vi "main_ctrl.vi"(8 "error in":errorcluster) -> (0 "error out":errorcluster caption="Error")   [LabVIEW 2013]
uses:
  <vilib>/Rock Robotics/WPI/DriverStation/WPI_DriverStationRobotMode2.ctl
  typedefs/fg_typedef.ctl
  typedefs/vision enable.ctl
  typedefs/vision data.ctl
  typedefs/subStates.ctl
  typedefs/singleUseSubstate.ctl
  <vilib>/Rock Robotics/WPI/Solenoid/WPI_SolenoidValue.ctl
  <vilib>/Rock Robotics/WPI/Compressor/WPI_CompressorGetSetRefNum.vi
  <vilib>/Rock Robotics/WPI/RobotDrive/WPI_RobotDriveGetSetRefNum.vi
  <vilib>/Rock Robotics/WPI/Solenoid/WPI_SolenoidSetEnum.vi
  <vilib>/Rock Robotics/WPI/RobotDrive/WPI_RobotDriveArcadeDrive_Standard(NoSaturation).vi
panel:
  out "Robot Mode":T1
  out "Vision SPI":u32
  out "Vision IPS":dbl
  out "Main IPS":dbl
  out "Main SPI":u32
  # "MAIN CONTROL"
  # "holds robot control code - dual parallel state machine"
  # "SPI: milliseconds per iteration\nIPS: iterations per second"
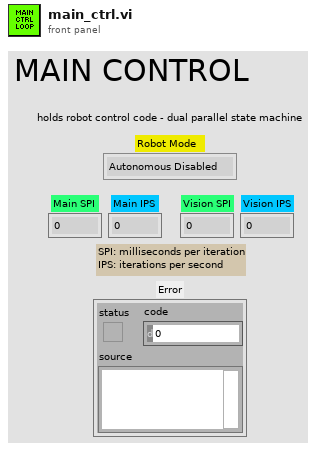
[diagram p1: front panel]
types:
  T1 = typedef "WPI_DriverStationRobotMode2.ctl" = enum16{"Autonomous Disabled", "Autonomous Enabled", "Teleop Disabled", "Teleop Enabled", "Timeout", "Finish", "Test Disabled", "Test Enabled"}
  T2 = typedef "vision data.ctl" = cluster{"x":dbl, "y":dbl, "area":dbl, "width":dbl, "height":dbl, "Hot Goal Present?":bool, "distance":dbl}
  T3 = typedef "vision enable.ctl" = enum16{"Enable", "Disable", "Stop"}
  T4 = typedef "fg_typedef.ctl" = enum16{"Get", "Set"}
  T5 = typedef "WPI_RobotDriveDevRef.ctl" = cluster{"DevStatus":errorcluster, "Motors[]":T6[], "Square Inputs":bool, "Max Output":dbl, "Isochronous":bool}
  T6 = typedef "WPI_MotorControlDeviceRef.ctl" = cluster{"DeviceStatus":errorcluster, "Type":enum16{"PWM", "CAN"}, "PWM":cluster{"Digital Module":T7, "PWM Channel":T8, "DeadBand":T9}, "CAN":cluster{"Device Number":u8, "Control Mode":T10, "Semaphore":T11, "Max Vout":dbl}, "Invert":bool, "TransformRef":T12, "InvTransformRef":T12}
  T7 = typedef "FPGA_TypedefDigitalModule.ctl" = enum16{"Digital Module 1", "Digital Module 2"}
  T8 = typedef "FPGA_DIOPWMChannel.ctl" = enum8{"PWM 1", "PWM 2", "PWM 3", "PWM 4", "PWM 5", "PWM 6", "PWM 7", "PWM 8", "PWM 9", "PWM 10", "Invalid"}
  T9 = typedef "WPI_PWMDeadband.ctl" = cluster{"Name":string, "maxPositivePwm":i32, "minPositivePwm":i32, "centerPwm":i32, "maxNegativePwm":i32, "minNegativePwm":i32, "angularRange":u16}
  T10 = typedef "WPI_CANJaguar_ControlMode.ctl" = enum8{"Percent VBus", "Current", "Speed", "Position", "Voltage"}
  T11 = typedef "Semaphore RefNum" = refnum<k1>
  T12 = typedef "WPI_PWMTransform_ConPane.ctl" = refnum<vi>
  T13 = typedef "WPI_SolenoidDevRef.ctl" = cluster{"DevStatus":errorcluster, "Solenoid Module":T14, "Forward Solenoid Channel":T15, "Reverse Solenoid Channel":T15}
  T14 = typedef "FPGA_TypedefSolenoidModule.ctl" = enum16{"Solenoid Module 1", "Solenoid Module 2"}
  T15 = typedef "WPI_SolenoidChannel.ctl" = enum8{"Solenoid 1", "Solenoid 2", "Solenoid 3", "Solenoid 4", "Solenoid 5", "Solenoid 6", "Solenoid 7", "Solenoid 8", "Invalid"}
  T16 = typedef "WPI_CompressorDevRef.ctl" = cluster{"DevStatus":errorcluster, "DigitalInputDevRef":T17, "RelayDevRef":T19}
  T17 = typedef "WPI_DigitalInputDevRef.ctl" = cluster{"DevStatus":errorcluster, "DIO Channel":T18, "Digital Module":T7}
  T18 = typedef "FPGA_DIOChannel.ctl" = enum8{"DIO 1", "DIO 2", "DIO 3", "DIO 4", "DIO 5", "DIO 6", "DIO 7", "DIO 8", "DIO 9", "DIO 10", "DIO 11", "DIO 12", "DIO 13", "DIO 14", "Invalid"}
  T19 = typedef "WPI_RelayDevRef.ctl" = cluster{"DevStatus":errorcluster, "Relay Channel":T20, "Digital Module":T7, "Relay Direction":T21}
  T20 = typedef "FPGA_DIORelayChannel.ctl" = enum8{"Relay 1", "Relay 2", "Relay 3", "Relay 4", "Relay 5", "Relay 6", "Relay 7", "Relay 8", "Invalid"}
  T21 = typedef "WPI_RelayDirection.ctl" = enum16{"Both directions", "Forward only", "Reverse only"}
  T22 = typedef "WPI_CameraDevRef.ctl" = cluster{"Camera Address":string, "CameraStatus":errorcluster, "Acquire Image Notifier":refnum<notifier>}
  T23 = typedef "IMAQ Image.ctl" = refnum<image>
  T24 = typedef "WPI_SolenoidValue.ctl" = enum16{"Off", "On", "Forward", "Reverse"}
  T25 = typedef "singleUseSubstate.ctl" = enum16{"null", "wait", "shift high", "shift low"}
  T26 = typedef "WPI_DriverStationDerivedRobotMode.ctl" = enum16{"Init", "Execute", "Stop"}
  T27 = typedef "subStates.ctl" = enum16{"null", "wait", "driver control", "auto", "manual override", "hold position", "rotate", "pickup", "pass", "load", "goto shoot", "shoot", "end"}
  T28 = typedef "Loop 2 Datatype.ctl" = cluster{"State":T27, "Waiting Loop":i32, "State to Wait For":i32, "Loop ID":i32, "Exit Value":i32, "Joystick Y":dbl, "Tune Speed":dbl}
  T29 = typedef "Loop 1 Datatype.ctl" = cluster{"State":T27, "Waiting Loop":i32, "State to Wait For":i32, "Loop ID":i32, "Exit Value":i32}
  T30 = typedef "Loop 3 Datatype.ctl" = cluster{"State":T27, "Waiting Loop":i32, "State to Wait For":i32, "Loop ID":i32, "Exit Value":i32, "Joystick Y":dbl, "Joystick Z":dbl}
  T31 = typedef "Loop 0 Datatype.ctl" = cluster{"State":T27, "Waiting Loop":i32, "State to Wait For":i32, "Loop ID":i32, "Exit Value":i32, "X Axis":dbl, "Y Axis":dbl, "Z Axis":dbl}
  T32 = typedef "Loop 4 Datatype.ctl" = cluster{"State":T27, "Waiting Loop":i32, "State to Wait For":i32, "Loop ID":i32, "Exit Value":i32}
  T33 = cluster{"Vision mSPI":u32, "Main mSPI":u32, "Dash mSPI":u32}
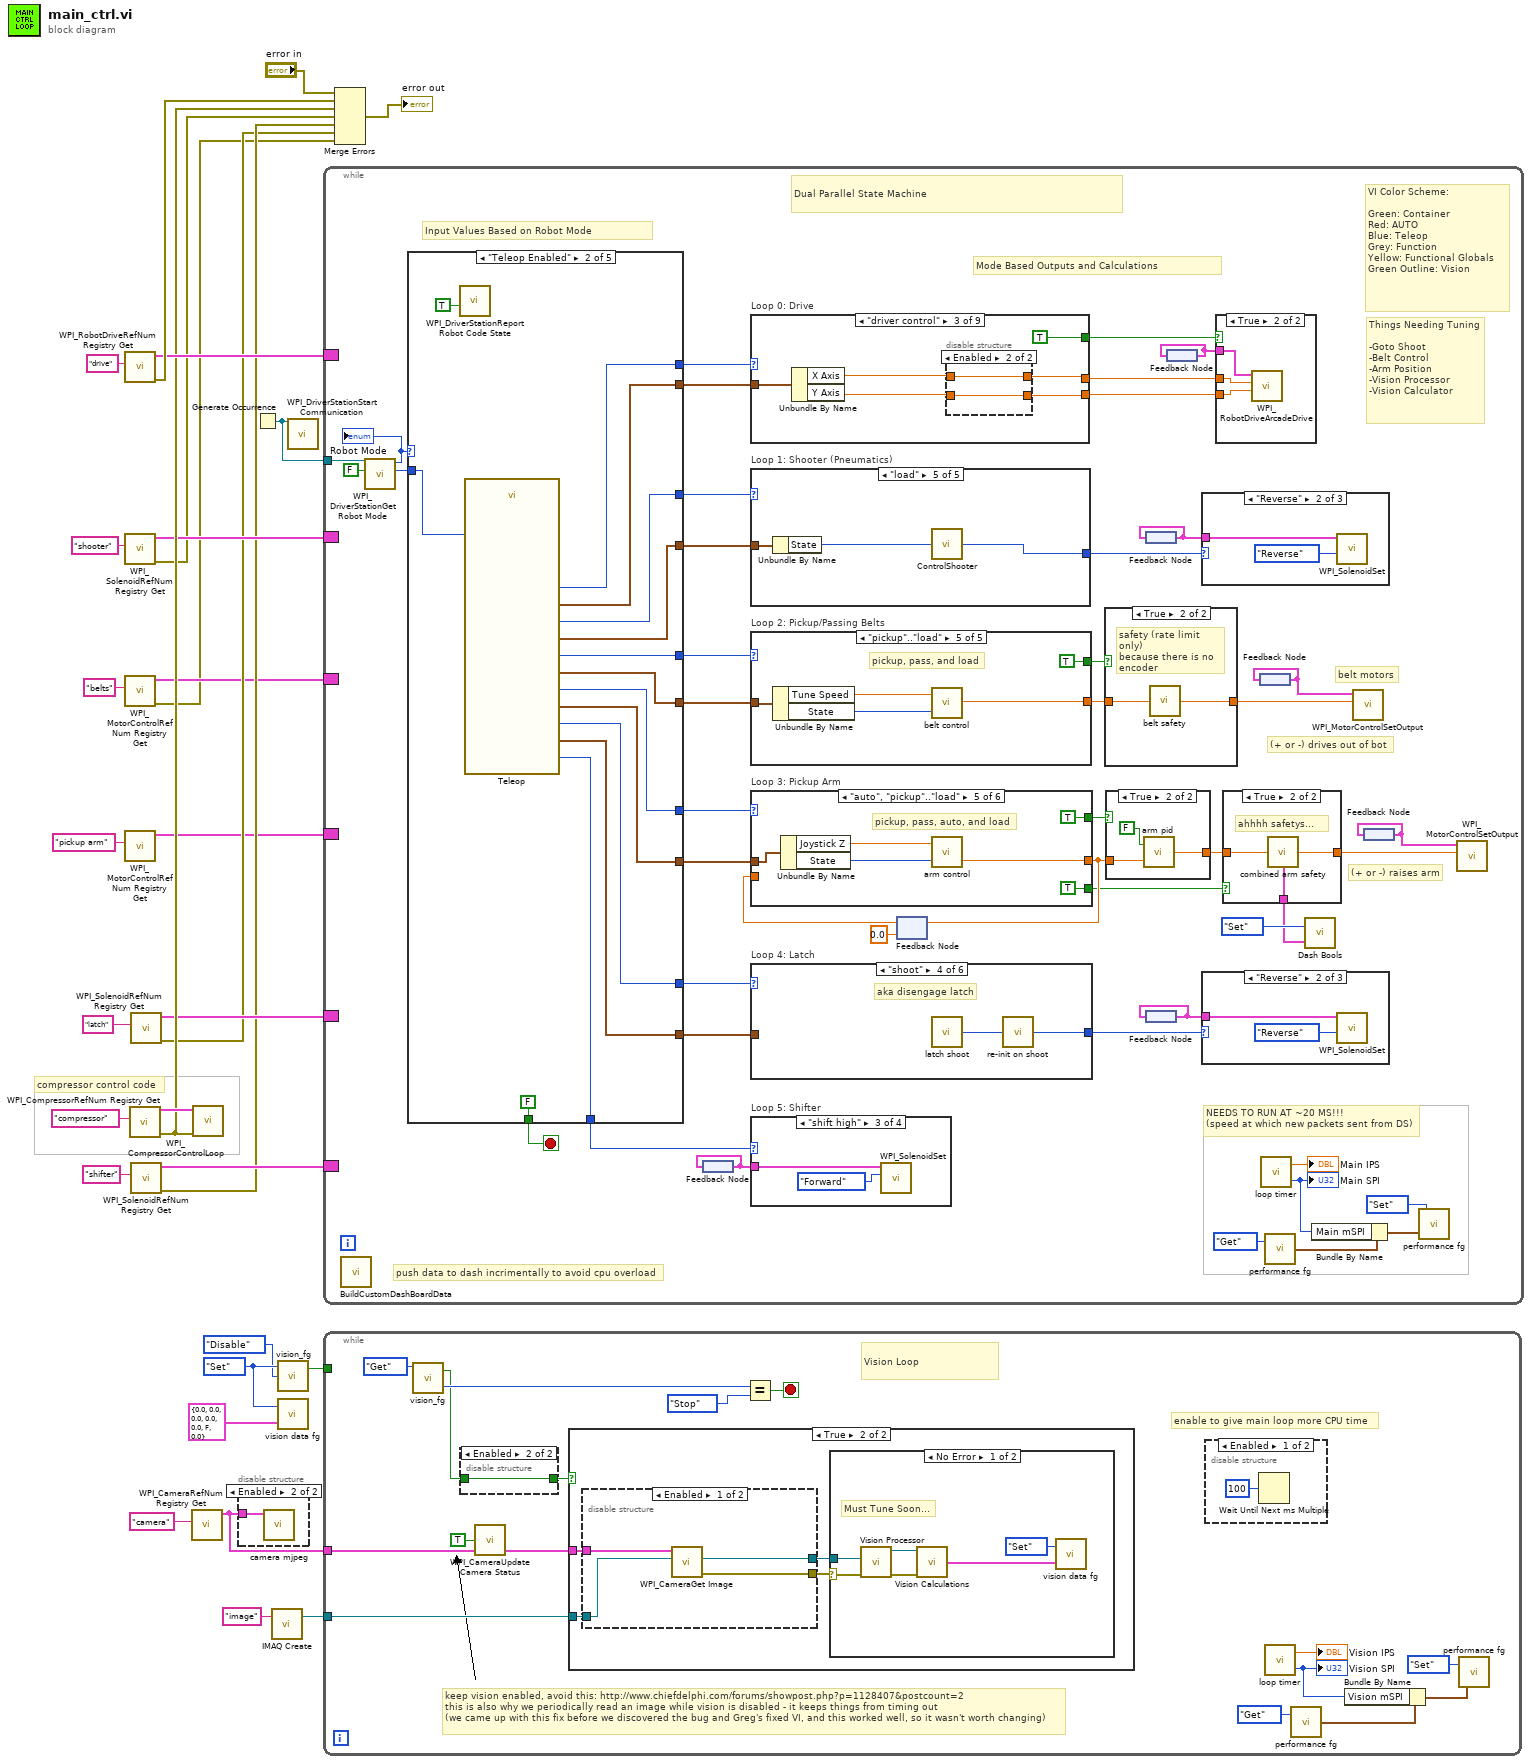
[diagram p0: block diagram]
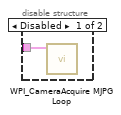
[diagram p2: hidden frame]
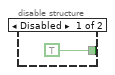
[diagram p3: hidden frame]
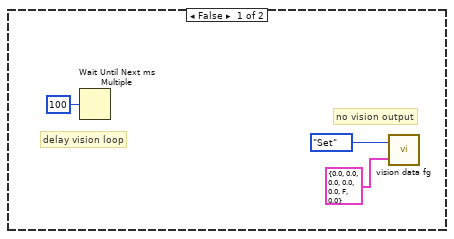
[diagram p5: hidden frame]
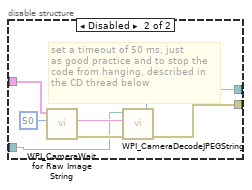
[diagram p7: hidden frame]
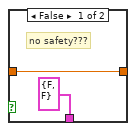
[diagram p9: hidden frame]
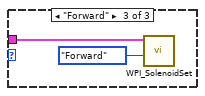
[diagram p12: hidden frame]
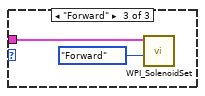
[diagram p14: hidden frame]
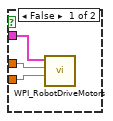
[diagram p15: hidden frame]
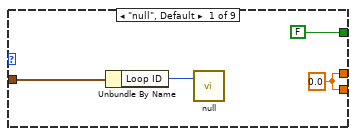
[diagram p16: hidden frame]
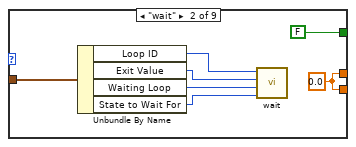
[diagram p17: hidden frame]
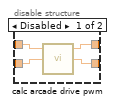
[diagram p18: hidden frame]
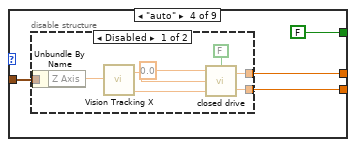
[diagram p19: hidden frame]
diagram:
  w19 = fg_typedef."Set" ("Enum")
  # "compressor control code"
  n1 = call <vilib>:"WPI_RobotDriveRefNum Registry Get.vi"("refnum name"="drive") -> ("error out"=w28:errorcluster, "RobotDriveDevRef"=w26:T5)  [unwired: 9 in]
  n2 = call <vilib>:"WPI_SolenoidRefNum Registry Get.vi"("refnum name"="shooter") -> ("error out"=w7:errorcluster, "SolenoidDevRef"=w11:T13)  [unwired: 9 in]
  n3 = call <vilib>:"WPI_MotorControlRefNum Registry Get.vi"("refnum name"="belts") -> ("error out"=w3:errorcluster, "MotorControlDevRef"=w5:T6)  [unwired: 9 in]
  n4 = call <vilib>:"WPI_MotorControlRefNum Registry Get.vi"("refnum name"="pickup arm") -> ("MotorControlDevRef"=w1:T6)  [unwired: 9 in, 1 out]
  n5 = call <vilib>:"WPI_CompressorRefNum Registry Get.vi"("refnum name"="compressor") -> ("error out"=w22:errorcluster, "CompressorDevRef"=w25:T16)  [unwired: 9 in]
  n6 = call <vilib>:"WPI_SolenoidRefNum Registry Get.vi"("refnum name"="latch") -> ("error out"=w6:errorcluster, "SolenoidDevRef"=w9:T13)  [unwired: 9 in]
  n7 = call <vilib>:"WPI_SolenoidRefNum Registry Get.vi"("refnum name"="shifter") -> ("error out"=w8:errorcluster, "SolenoidDevRef"=w24:T13)  [unwired: 9 in]
  n8 = call <vilib>:"WPI_CameraRefNum Registry Get.vi"("refnum name"="camera") -> ("CameraDevRef"=w16:T22)  [unwired: 9 in, 1 out]
  n9 = call <vilib>:"WPI_CompressorControlLoop.vi"("error in (no error)"=w22, "CompressorDevRef"=w25) -> ()  [unwired: 10 in]
  n10 = disable-structure shown="Enabled" {
    disable-tunnel: w16 -> [w32 w33]
    frame Disabled {
      n11 = call <vilib>:"WPI_CameraAcquire MJPG Loop.vi"("CameraDevRef"=w32) -> ()  [unwired: 11 in]
    }
    frame Enabled {
      n12 = call "camera mjpeg.vi"("CameraDevRef"=w33) -> ()  [unwired: 11 in]
    }
  }
  n13 = Generate Occurrence() -> (w14:refnum<k4>)
  n14 = call "IMAQ Create"("Image Name"="image") -> ("New Image"=w21:T23)  [unwired: 4 in, 1 out]
  n15 = call "vision_fg.vi"("Action"=vision_enable."Disable", "Menu"=w19) -> ("Enabled?"=w20:bool)  [unwired: 1 in, 1 out]
  n16 = call "vision data fg.vi"("Input"=T2 {"x"=0.0, "y"=0.0, "area"=0.0, "width"=0.0, "height"=0.0, "Hot Goal Present?"=FALSE, "distance"=0.0} ("Cluster"), "Menu"=w19) -> ()  [unwired: 1 out]
  n17 = call <vilib>:"WPI_DriverStationStart Communication.vi"("occurrence"=w14) -> ()  [unwired: 11 in]
  n18 = while {
    tunnel: w14 -> [w54]
    border: w26 -> [_]
    border: w24 -> [_]
    border: w11 -> [_]
    border: w9 -> [_]
    border: w5 -> [_]
    border: w1 -> [_]
    stop <- w75 stop-if-true
    # "push data to dash incrimentally to avoid cpu overload"
    # "Things Needing Tuning\n\n-Goto Shoot\n-Belt Control\n-Arm Position\n-Vision Processor\n-Vision Calculator"
    # "(+ or -) raises arm"
    # "(+ or -) drives out of bot"
    # "belt motors"
    # "VI Color Scheme:\n\nGreen: Container\nRed: AUTO\nBlue: Teleop\nGrey: Function\nYellow: Functional Globals\nGreen Outline: Vision"
    # "Input Values Based on Robot Mode"
    # "Mode Based Outputs and Calculations"
    # "NEEDS TO RUN AT ~20 MS!!!\n(speed at which new packets sent from DS)"
    # "Dual Parallel State Machine"
    n19 = call "BuildCustomDashBoardData.vi"() -> ()  [unwired: 12 in]
    n20 = call <vilib>:"WPI_DriverStationGet Robot Mode.vi"("Finish"=FALSE, "DS Occurrence"=w54) -> ("Call Context"=w53:T26, "Robot Mode"=w52:T1)  [unwired: 8 out]
    "Robot Mode" <- w52
    n21 = case shown="\"Teleop Enabled\"" w52 {
      tunnel: [w265 w282 w284 w290 w296] -> w56
      tunnel: w53 -> [w256 w278 _ _ _]
      tunnel: [w263 w281 w284 w290 w296] -> w77
      tunnel: [w257 w279 singleUseSubstate."null" ("SubState 5") singleUseSubstate."null" ("SubState 5") singleUseSubstate."null" ("SubState 5")] -> w76
      tunnel: [FALSE FALSE FALSE FALSE TRUE] -> w75
      tunnel: [w267 w277 w284 w290 w296] -> w68
      tunnel: [w266 w276 _ _ _] -> w69
      tunnel: [w264 w275 _ _ _] -> w67
      tunnel: [w262 w274 _ _ _] -> w66
      tunnel: [w260 w273 _ _ _] -> w64
      tunnel: [w258 w272 _ _ _] -> w63
      tunnel: [w259 w271 w284 w290 w296] -> w62
      tunnel: [w261 w270 w284 w290 w296] -> w61
      frame "Autonomous Enabled" {
        n22 = call <vilib>:"WPI_DriverStationReport Robot Code State.vi"("Autonomous"=TRUE) -> ()  [unwired: 10 in, 1 out]
        n23 = call "Autonomous.vi"("Call Context"=w256) -> ("SubState 2"=w263:T27, "Loop 2 Data"=w262:T28, "SubState 1"=w265:T27, "Loop 1 Data"=w264:T29, "Loop 3 Data"=w260:T30, "SubState 0"=w267:T27, "SubState 3"=w261:T27, "Loop 0 Data"=w266:T31, "Loop 4 Data"=w258:T32, "SubState 4"=w259:T27, "SubState 5"=w257:T25)
      }
      frame "Teleop Enabled" {
        n24 = call <vilib>:"WPI_DriverStationReport Robot Code State.vi"("TeleOp"=TRUE) -> ()  [unwired: 10 in, 1 out]
        n25 = call "Teleop.vi"("Call Context"=w278) -> ("SubState 3"=w270:T27, "SubState 4"=w271:T27, "SubState 5"=w279:T25, "Loop 3 Data"=w273:T30, "Loop 4 Data"=w272:T32, "SubState 0"=w277:T27, "Loop 1 Data"=w275:T29, "Loop 0 Data"=w276:T31, "SubState 1"=w282:T27, "Loop 2 Data"=w274:T28, "SubState 2"=w281:T27)  [unwired: 8 in]
      }
      frame "Autonomous Disabled", "Teleop Disabled", "Timeout" {
        w284 = subStates."null" ("SubState 0")
        # "set all loops to null"
        # "make sure to disable vision\nwe don't need it here"
        # "robot disabled, timeout"
        n26 = call <vilib>:"WPI_DriverStationReport Robot Code State.vi"("Disabled"=TRUE) -> ()  [unwired: 10 in, 1 out]
        n27 = call "vision_fg.vi"("Action"=vision_enable."Disable", "Menu"=fg_typedef."Set") -> ()  [unwired: 1 in, 2 out]
      }
      frame "Test Disabled", "Test Enabled" {
        w290 = subStates."null" ("SubState 0")
        # "set all loops to null"
        # "make sure to disable vision\nwe don't need it here"
        # "test, unused"
        n28 = call <vilib>:"WPI_DriverStationReport Robot Code State.vi"("Test"=TRUE) -> ()  [unwired: 10 in, 1 out]
        n29 = call "vision_fg.vi"("Action"=vision_enable."Disable", "Menu"=fg_typedef."Set") -> ()  [unwired: 1 in, 2 out]
      }
      frame "Finish" {
        w296 = subStates."end"  # Stop All Loops
        # "stop the while loop"
        # "stop DS comms"
        # "stop vision loop"
        n30 = call <vilib>:"WPI_DriverStationStop Communication.vi"("StopCommunication"=TRUE) -> ()  [unwired: 10 in, 1 out]
        n31 = call "vision_fg.vi"("Action"=vision_enable."Stop", "Menu"=fg_typedef."Set") -> ()  [unwired: 1 in, 2 out]
      }
    }
    n32 = feedback #1() -> (w65:T13)
    n33 = feedback-in #1(w65) -> ()
    n34 = case "Loop 0: Drive" shown="\"driver control\"" w68 {
      tunnel: w69 -> [w107 w111 w121 w128 w145 w152 _ _ w168]
      tunnel: [w105 w109 w117 w130 w142 w154 w157 w162 w164] -> w59
      tunnel: [w105 w109 w116 w129 w141 w153 w156 w162 w163] -> w58
      tunnel: [FALSE FALSE TRUE FALSE FALSE FALSE FALSE FALSE FALSE] -> w60
      frame "null", Default {
        w105 = 0.0 ("X Axis")
        n35 = Unbundle By Name(w107) -> ("Loop ID"=w108:i32)
        n36 = call "null.vi"("This Loop ID"=w108) -> ()  [unwired: 2 in]
      }
      frame "wait" {
        w109 = 0.0 ("X Axis")
        n37 = Unbundle By Name(w111) -> ("Loop ID"=w115:i32, "Exit Value"=w114:i32, "Waiting Loop"=w113:i32, "State to Wait For"=w112:i32)
        n38 = call "wait.vi"("State to wait for"=w112, "Waiting Loop ID"=w113, "time (ms)"=w114, "Current Loop ID"=w115) -> ()  [unwired: 1 out]
      }
      frame "driver control" {
        n39 = Unbundle By Name(w121) -> ("X Axis"=w119:dbl, "Y Axis"=w118:dbl)
        n40 = disable-structure shown="Enabled" {
          disable-tunnel: w119 -> [w125 w127]
          disable-tunnel: w118 -> [w124 w126]
          disable-tunnel: [w123 w127] -> w117
          disable-tunnel: [w122 w126] -> w116
          frame Disabled {
            n41 = call "calc arcade drive pwm.vi"("Y axis value"=w124, "X axis value"=w125) -> ("Right Speed"=w122:dbl, "Left Speed"=w123:dbl)  [unwired: 1 in, 1 out]
          }
          frame Enabled {
          }
        }
      }
      frame "auto" {
        n42 = disable-structure shown="Disabled" {
          disable-tunnel: [w139 _] -> w130
          disable-tunnel: [w138 _] -> w129
          disable-tunnel: w128 -> [w134 _]
          frame Disabled {
            n43 = Unbundle By Name(w134) -> ("Z Axis"=w132:dbl)
            n44 = call "Vision Tracking X.vi"("Tweak"=w132) -> ("right speed"=w133:dbl, "left speed"=w136:dbl)
            n45 = call "closed drive.vi"("Acrade Drive?"=FALSE, "Y axis value (Left)"=w136, "X axis value (Right)"=w133, "Threshold (.4)"=0.0 ("Threshold")) -> ("right"=w138:dbl, "left"=w139:dbl)
          }
          frame Enabled {
            # "rotates toward target"
            # "not in use this year"
          }
        }
      }
      frame "hold position" {
        n46 = Unbundle By Name(w145) -> ("X Axis"=w144:dbl, "Y Axis"=w143:dbl)
        n47 = call "closed drive.vi"("Acrade Drive?"=TRUE, "Y axis value (Left)"=w143, "X axis value (Right)"=w144) -> ("right"=w141:dbl, "left"=w142:dbl)  [unwired: 1 in]
      }
      frame "rotate" {
        # "use these to carry actual information because this is\nfor autonomous only so there will not be joystick input"
        n48 = Unbundle By Name(w152) -> ("X Axis"=w151:dbl, "Y Axis"=w150:dbl)
        n49 = call "rotate.vi"("Angle"=w151, "Rate"=w150) -> ("finished?"=w147:bool, "left speed"=w154:dbl, "right speed"=w153:dbl)
        n50 = call "states FG.vi"("exit in"=w147, "menu (get)"=enum16{"set", "get"}."set", "Loop ID"=0) -> ()  [unwired: 5 in, 4 out]
      }
      frame "goto shoot" {
        # "consider implimenting closed hold with drive"
        n51 = call "vision data fg.vi"("Menu"=fg_typedef."Get") -> ("Output"=w158:T2)  [unwired: 1 in]
        n52 = call "goto location.vi"("Image Data"=w158) -> ("left speed"=w157:dbl, "right speed"=w156:dbl)
      }
      frame "end" {
        w162 = 0.0 ("X Axis")
      }
      frame "manual override" {
        n53 = Unbundle By Name(w168) -> ("X Axis"=w167:dbl, "Y Axis"=w166:dbl)
        n54 = expression code="x/2"(w167) -> (w164:dbl)
        n55 = expression code="x/2"(w166) -> (w163:dbl)
      }
    }
    n56 = case "Loop 1: Shooter (Pneumatics)" shown="\"load\"" w56 {
      tunnel: w67 -> [w242 w245 _ _ w254]
      tunnel: [WPI_SolenoidValue."Off" ("Value") WPI_SolenoidValue."Off" ("Value") WPI_SolenoidValue."Off" ("Value") WPI_SolenoidValue."Off" ("Value") w252] -> w51
      frame "null", Default {
        n57 = Unbundle By Name(w242) -> ("Loop ID"=w243:i32)
        n58 = call "null.vi"("This Loop ID"=w243) -> ()  [unwired: 2 in]
      }
      frame "wait" {
        n59 = Unbundle By Name(w245) -> ("Loop ID"=w249:i32, "Exit Value"=w248:i32, "Waiting Loop"=w247:i32, "State to Wait For"=w246:i32)
        n60 = call "wait.vi"("State to wait for"=w246, "Waiting Loop ID"=w247, "time (ms)"=w248, "Current Loop ID"=w249) -> ()  [unwired: 1 out]
      }
      frame "driver control" {
      }
      frame "manual override" {
      }
      frame "load" {
        n61 = Unbundle By Name(w254) -> ("State"=w253:T27)
        n62 = call "ControlShooter.vi"("State"=w253) -> ("To Shooter\nSolenoid Loop"=w252:T24)
      }
    }
    n63 = case "Loop 2: Pickup/Passing Belts" shown="\"pickup\"..\"load\"" w77 {
      tunnel: w66 -> [w221 w224 w231 w235 w240]
      tunnel: [0.0 ("output") 0.0 ("output") w230 w233 w237] -> w37
      tunnel: [FALSE FALSE TRUE FALSE TRUE] -> w38
      frame "null", Default {
        n64 = Unbundle By Name(w221) -> ("Loop ID"=w220:i32)
        n65 = call "null.vi"("This Loop ID"=w220) -> ()  [unwired: 2 in]
      }
      frame "wait" {
        n66 = Unbundle By Name(w224) -> ("Loop ID"=w228:i32, "Exit Value"=w227:i32, "Waiting Loop"=w226:i32, "State to Wait For"=w225:i32)
        n67 = call "wait.vi"("State to wait for"=w225, "Waiting Loop ID"=w226, "time (ms)"=w227, "Current Loop ID"=w228) -> ()  [unwired: 1 out]
      }
      frame "driver control" {
        n68 = Unbundle By Name(w231) -> ("Joystick Y"=w230:dbl)
      }
      frame "manual override" {
        n69 = Unbundle By Name(w235) -> ("Joystick Y"=w234:dbl)
        n70 = expression code="x/2"(w234) -> (w233:dbl)
      }
      frame "pickup".."load" {
        # "pickup, pass, and load"
        n71 = Unbundle By Name(w240) -> ("Tune Speed"=w239:dbl, "State"=w238:T27)
        n72 = call "belt control.vi"("State"=w238, "Joystick Z"=w239) -> ("output"=w237:dbl)
      }
    }
    n73 = case "Loop 4: Latch" shown="\"shoot\"" w62 {
      tunnel: w63 -> [w171 w173 _ _ _ _]
      tunnel: [WPI_SolenoidValue."Off" ("Value") WPI_SolenoidValue."Off" ("Value") WPI_SolenoidValue."Off" ("Value") w179 WPI_SolenoidValue."Forward" ("Value") WPI_SolenoidValue."Reverse" ("Value")] -> w48
      frame "null", Default {
        n74 = Unbundle By Name(w171) -> ("Loop ID"=w170:i32)
        n75 = call "null.vi"("This Loop ID"=w170) -> ()  [unwired: 2 in]
      }
      frame "wait" {
        n76 = Unbundle By Name(w173) -> ("Loop ID"=w177:i32, "Exit Value"=w176:i32, "Waiting Loop"=w175:i32, "State to Wait For"=w174:i32)
        n77 = call "wait.vi"("State to wait for"=w174, "Waiting Loop ID"=w175, "time (ms)"=w176, "Current Loop ID"=w177) -> ()  [unwired: 1 out]
      }
      frame "driver control" {
      }
      frame "shoot" {
        # "aka disengage latch"
        n78 = call "latch shoot.vi"() -> ("Latch"=w180:T24)
        n79 = call "re-init on shoot.vi"("Relay Value"=w180) -> ("Value"=w179:T24)
      }
      frame "auto" {
        # "aka engage"
      }
      frame "manual override" {
        # "unsafely shoot"
      }
    }
    n80 = case "Loop 5: Shifter" shown="\"shift high\"" w76 {
      tunnel: w65 -> [_ _ w215 w216]
      frame "null", Default {
      }
      frame "wait" {
      }
      frame "shift high" {
        n81 = call-poly <vilib>:"WPI_SolenoidSet.vi"("Value"=WPI_SolenoidValue."Forward", "SolenoidDevRef"=w215) -> ()  [unwired: 8 in, 2 out]
      }
      frame "shift low" {
        n82 = call-poly <vilib>:"WPI_SolenoidSet.vi"("Value"=WPI_SolenoidValue."Reverse", "SolenoidDevRef"=w216) -> ()  [unwired: 8 in, 2 out]
      }
    }
    n83 = feedback #2(0.0 ("output")) -> (w43:dbl)
    n84 = case "Loop 3: Pickup Arm" shown="\"auto\", \"pickup\"..\"load\"" w61 {
      tunnel: w64 -> [w187 w191 w198 w204 w210 _]
      tunnel: [FALSE FALSE FALSE FALSE TRUE TRUE] -> w45
      tunnel: [0.0 ("output") 0.0 ("output") w197 w202 w206 w212] -> w44
      tunnel: w43 -> [_ _ _ _ _ w212]
      tunnel: [TRUE TRUE TRUE FALSE TRUE TRUE] -> w41
      frame "null", Default {
        n85 = Unbundle By Name(w187) -> ("Loop ID"=w186:i32)
        n86 = call "null.vi"("This Loop ID"=w186) -> ()  [unwired: 2 in]
      }
      frame "wait" {
        n87 = Unbundle By Name(w191) -> ("Loop ID"=w195:i32, "Exit Value"=w194:i32, "Waiting Loop"=w193:i32, "State to Wait For"=w192:i32)
        n88 = call "wait.vi"("State to wait for"=w192, "Waiting Loop ID"=w193, "time (ms)"=w194, "Current Loop ID"=w195) -> ()  [unwired: 1 out]
      }
      frame "driver control" {
        n89 = Unbundle By Name(w198) -> ("Joystick Y"=w197:dbl)
      }
      frame "manual override" {
        n90 = Unbundle By Name(w204) -> ("Joystick Y"=w203:dbl)
        n91 = expression code="x/2"(w203) -> (w202:dbl)
      }
      frame "auto", "pickup".."load" {
        # "pickup, pass, auto, and load"
        n92 = Unbundle By Name(w210) -> ("Joystick Z"=w208:dbl, "State"=w207:T27)
        n93 = call "arm control.vi"("State"=w207, "Z Axis (Tuning)"=w208) -> ("setpoint"=w206:dbl)
      }
      frame "hold position" {
      }
    }
    n94 = feedback-in #2(w44) -> ()
    n95 = case shown="True" w38 {
      tunnel: w37 -> [w79 w81]
      tunnel: [w79 w80] -> w36
      frame False {
        # "no safety"
      }
      frame True {
        # "safety (rate limit only)\nbecause there is no \nencoder"
        n96 = call "belt safety.vi"("Input"=w81) -> ("Safe Output"=w80:dbl)
      }
    }
    n97 = case shown="True" w45 {
      tunnel: w44 -> [w87 w90]
      tunnel: [w87 w89] -> w40
      frame False {
        # "open loop"
      }
      frame True {
        n98 = call "arm pid.vi"("Setpoint"=w90, "Autotune?"=FALSE) -> ("Output"=w89:dbl)
      }
    }
    n99 = feedback #3() -> (w50:T13)
    n100 = feedback-in #3(w50) -> ()
    n101 = feedback #4() -> (w49:T13)
    n102 = feedback-in #4(w49) -> ()
    n103 = feedback #5() -> (w57:T5)
    n104 = feedback-in #5(w57) -> ()
    n105 = case shown="\"Reverse\"" w51 {
      tunnel: w50 -> [_ w95 w97]
      frame "Off", Default {
      }
      frame "Reverse" {
        n106 = call-poly <vilib>:"WPI_SolenoidSet.vi"("Value"=WPI_SolenoidValue."Reverse", "SolenoidDevRef"=w95) -> ()  [unwired: 8 in, 2 out]
      }
      frame "Forward" {
        n107 = call-poly <vilib>:"WPI_SolenoidSet.vi"("Value"=WPI_SolenoidValue."Forward", "SolenoidDevRef"=w97) -> ()  [unwired: 8 in, 2 out]
      }
    }
    n108 = case shown="\"Reverse\"" w48 {
      tunnel: w49 -> [_ w91 w93]
      frame "Off", Default {
      }
      frame "Reverse" {
        n109 = call-poly <vilib>:"WPI_SolenoidSet.vi"("Value"=WPI_SolenoidValue."Reverse", "SolenoidDevRef"=w91) -> ()  [unwired: 8 in, 2 out]
      }
      frame "Forward" {
        n110 = call-poly <vilib>:"WPI_SolenoidSet.vi"("Value"=WPI_SolenoidValue."Forward", "SolenoidDevRef"=w93) -> ()  [unwired: 8 in, 2 out]
      }
    }
    n111 = case shown="True" w60 {
      tunnel: w59 -> [w100 w104]
      tunnel: w58 -> [w99 w103]
      tunnel: w57 -> [w101 w102]
      frame False {
        n112 = call <vilib>:"WPI_RobotDriveMotors.vi"("RightSpeed"=w99, "LeftSpeed"=w100, "RobotDriveDevRef"=w101) -> ()  [unwired: 6 in, 3 out]
      }
      frame True {
        n113 = call-poly <vilib>:"WPI_RobotDriveArcadeDrive.vi"("Y axis value"=w103, "X axis value"=w104, "RobotDriveDevRef"=w102) -> ()  [unwired: 6 in, 3 out]
      }
    }
    n114 = case shown="True" w41 {
      tunnel: w40 -> [w83 w86]
      tunnel: [w83 w85] -> w39
      tunnel: [cluster{"Arm Safety":bool, "Arm Limit":bool} {"Arm Safety"=FALSE, "Arm Limit"=FALSE} ("Input") w84] -> w34
      frame False {
        # "no safety???"
      }
      frame True {
        # "ahhhh safetys..."
        n115 = call "combined arm safety.vi"("Input"=w86) -> ("Safe Output"=w85:dbl, "Safety"=w84:cluster{"Arm Safety":bool, "Arm Limit":bool})  [unwired: 13 in]
      }
    }
    n116 = feedback #6() -> (w47:T6)
    n117 = feedback-in #6(w47) -> ()
    n118 = call "loop timer.vi"() -> ("IPS"=→"Main IPS":dbl, "SPI"=w74:u32)  [unwired: 1 in]
    "Main SPI" <- w74
    n119 = call "performance fg.vi"("Menu"=fg_typedef."Get") -> ("Output"=w71:T33)  [unwired: 1 in]
    n120 = call "Dash Bools.vi"("Input"=w34, "Menu"=fg_typedef."Set") -> ()  [unwired: 1 out]
    n121 = Bundle By Name(cluster=w71, "Main mSPI"=w74) -> (w70:T33)
    n122 = call <vilib>:"WPI_MotorControlSetOutput.vi"("Output"=w36, "MotorControlDevRef"=w47) -> ()  [unwired: 7 in, 3 out]
    n123 = feedback #7() -> (w46:T6)
    n124 = feedback-in #7(w46) -> ()
    n125 = call "performance fg.vi"("Input"=w70, "Menu"=fg_typedef."Set") -> ()  [unwired: 1 out]
    n126 = call <vilib>:"WPI_MotorControlSetOutput.vi"("Output"=w39, "MotorControlDevRef"=w46) -> ()  [unwired: 7 in, 3 out]
  }
  n127 = while {
    tunnel: w21 -> [w315]
    tunnel: w16 -> [w314]
    tunnel: w20 -> [_]
    stop <- w316 stop-if-true
    # "keep vision enabled, avoid this: http://www.chiefdelphi.com/forums/showpost.php?p=1128407&postcount=2\nthis is also why we periodically read an image while vision is disabled - it keeps things from timing out\n(we came up with this fix before we discovered the bug and Greg's fixed VI, and this worked well, so it wasn't worth changing)"
    # "enable to give main loop more CPU time"
    # "Vision Loop"
    n128 = call "vision_fg.vi"("Menu"=fg_typedef."Get" ("Enum")) -> ("State Out"=w310:T3, "Enabled?"=w301:bool)  [unwired: 2 in]
    n129 = disable-structure shown="Enabled" {
      disable-tunnel: [TRUE w318] -> w302
      disable-tunnel: w301 -> [_ w318]
      frame Disabled {
      }
      frame Enabled {
      }
    }
    n130 = call <vilib>:"WPI_CameraUpdate Camera Status.vi"("CameraDevRef In"=w314, "Enable Vision"=TRUE) -> ("CameraDevRef Out"=w313:T22)  [unwired: 3 in]
    n131 = case shown="True" w302 {
      tunnel: w315 -> [_ w326]
      tunnel: w313 -> [_ w325]
      frame False {
        # "no vision output"
        # "delay vision loop"
        n132 = Wait Until Next ms Multiple(millisecond multiple=u32 100) -> ()  [unwired: 1 out]
        n133 = call "vision data fg.vi"("Input"=T2 {"x"=0.0, "y"=0.0, "area"=0.0, "width"=0.0, "height"=0.0, "Hot Goal Present?"=FALSE, "distance"=0.0} ("Cluster"), "Menu"=fg_typedef."Set" ("Enum")) -> ()  [unwired: 1 out]
      }
      frame True {
        n134 = disable-structure shown="Enabled" {
          disable-tunnel: w326 -> [w335 w339]
          disable-tunnel: w325 -> [w336 w341]
          disable-tunnel: [w334 w338] -> w324
          disable-tunnel: [w333 w337] -> w323
          frame Enabled {
            n135 = call <vilib>:"WPI_CameraGet Image.vi"("Image"=w335, "CameraDevRef"=w336) -> ("error out"=w333:errorcluster, "Image Out"=w334:T23)  [unwired: 7 in, 1 out]
          }
          frame Disabled {
            # "set a timeout of 50 ms, just\nas good practice and to stop the \ncode from hanging, described in \nthe CD thread below"
            n136 = call <vilib>:"WPI_CameraWait for Raw Image String.vi"("Timeout in ms (-1)"=50, "CameraDevRef"=w341) -> ("error out"=w343:errorcluster, "String"=w342:string)  [unwired: 3 in, 5 out]
            n137 = call <vilib>:"WPI_CameraDecodeJPEGString.vi"("error in"=w343, "Compressed Image"=w342, "Image In"=w339) -> ("error out"=w337:errorcluster, "Image Out"=w338:T23)  [unwired: 3 out]
          }
        }
        n138 = case shown="No Error" w323 {
          selector: w323 -> [w331 _]
          tunnel: w324 -> [w330 _]
          frame No Error {
            # "Must Tune Soon..."
            n139 = call "Vision Processor.vi"("error in"=w331, "Image In"=w330) -> ("error out"=w328:errorcluster, "Image Out"=w329:T23)  [unwired: 5 in]
            n140 = call "Vision Calculations.vi"("Image In"=w329, "error in"=w328) -> ("Vision Data"=w327:T2)  [unwired: 3 in]
            n141 = call "vision data fg.vi"("Input"=w327, "Menu"=fg_typedef."Set" ("Enum")) -> ()  [unwired: 1 out]
          }
          frame Error {
          }
        }
      }
    }
    n142 = Equal?(x=w310, y=vision_enable."Stop") -> (x = y?=w316:bool)
    n143 = disable-structure shown="Enabled" {
      frame Enabled {
        n144 = Wait Until Next ms Multiple(millisecond multiple=u32 100) -> ()  [unwired: 1 out]
      }
      frame Disabled {
      }
    }
    n145 = call "loop timer.vi"() -> ("IPS"=→"Vision IPS":dbl, "SPI"=w308:u32)  [unwired: 1 in]
    "Vision SPI" <- w308
    n146 = call "performance fg.vi"("Menu"=fg_typedef."Get") -> ("Output"=w306:T33)  [unwired: 1 in]
    n147 = Bundle By Name(cluster=w306, "Vision mSPI"=w308) -> (w305:T33)
    n148 = call "performance fg.vi"("Input"=w305, "Menu"=fg_typedef."Set") -> ()  [unwired: 1 out]
  }
  n149 = Merge Errors("error in", w28, w22, w7, w8, w6, w3) -> (→"error out":errorcluster)
